vi "SendMessage_Cluster.vi"(6 "timeout in ms (-1)":i32=-1, 8 "error in":errorcluster, 10 "message":T1, 11 "message ref in":refnum<class "CLM_LocalMessage.lvclass">) -> (0 "error out":errorcluster, 3 "message ref out":refnum<class "CLM_LocalMessage.lvclass">, 4 "timed out?":bool)   [LabVIEW 2013, in "CLM_LocalMessage.lvclass"]
uses:
  CLM_LocalMessage.lvclass
  Message.ctl
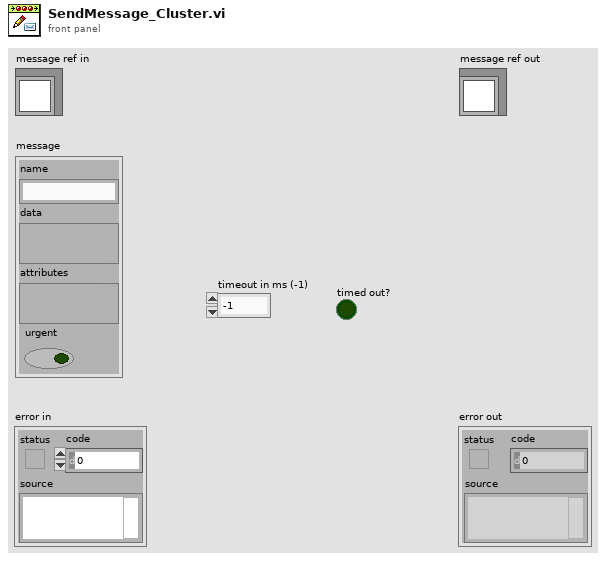
[diagram p1: front panel]
types:
  T1 = typedef "CLM_LocalMessage.lvclass/Message.ctl" = cluster{"name":string, "data":variant, "attributes":variant, "urgent":bool}
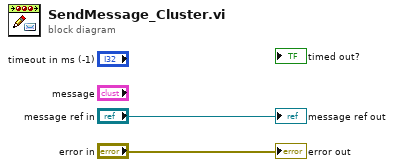
[diagram p0: block diagram]
diagram:
  "error out" <- "error in"
  "message ref out" <- "message ref in"
